vi "Gaussian surface with offset model.vi"(3 "output control":T1, 4 "data":variant, 5 "X":dbl[](array[numeric]), 6 "a":dbl[](array[numeric])) -> (0 "error out":errorcluster, 1 "f'(X,a)":dbl[][](array[numeric]), 2 "f(X,a)":dbl[](array[numeric]))   [LabVIEW 2023]
doc: "Gaussian surface with offset model"
uses:
  <vilib>/gmath/NumericalOptimization/LM_output select.ctl
  <vilib>/Utility/error.llb/Error Cluster From Error Code.vi
  <vilib>/Native 3D Graph/xcontrol/3DPC_SurfacePlot.xctl
  <vilib>/Native 3D Graph/classes/Base Datatype.lvclass
  <vilib>/ErrorRing/Error Ring.xnode
  <vilib>/gmath/NI_Gmath.lvlib
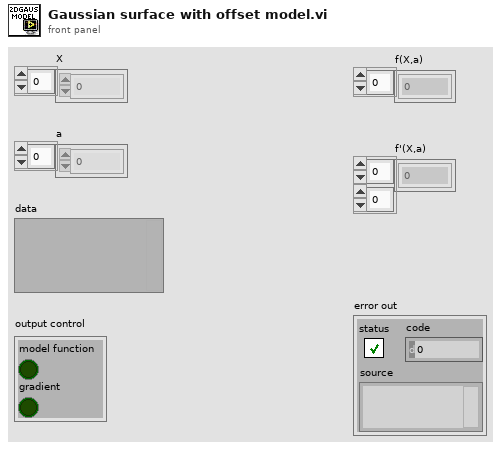
[diagram p1: front panel]
types:
  T1 = typedef "NI_Gmath.lvlib/LM_output select.ctl" = cluster{"model function":bool, "gradient":bool}
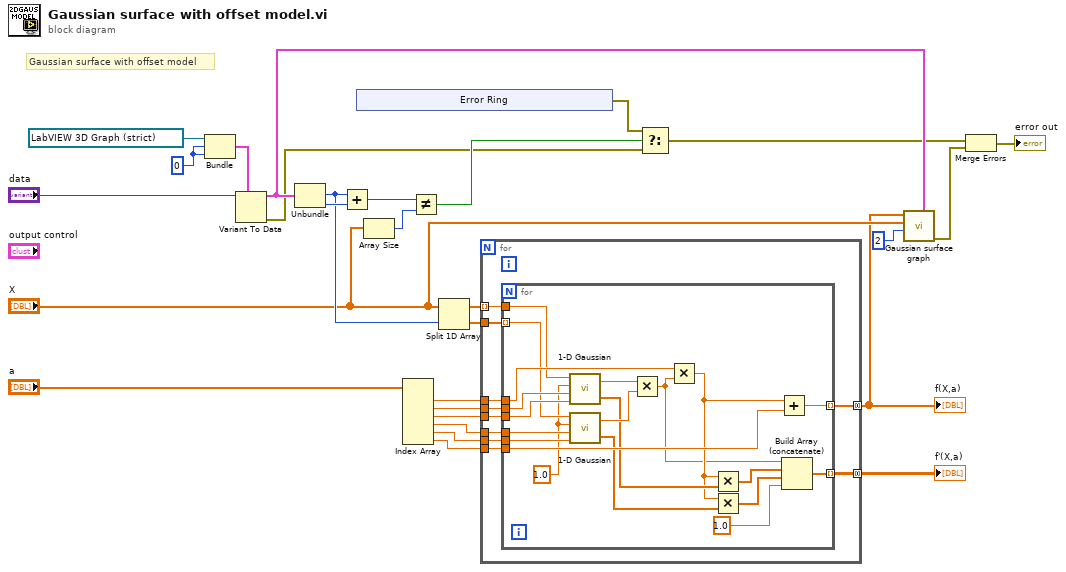
[diagram p0: block diagram]
diagram:
  w23 = 0
  # "Gaussian surface with offset model"
  n1 = Bundle("3D Surface Graph"=refnum<vi> refnum, w23, w23) -> (w15:cluster{"3D Surface Graph":refnum<vi>, i32, i32})  [unwired: 1 out]
  n2 = Variant To Data(type=w15, Variant="data") -> (data=w12:cluster{"3D Surface Graph":refnum<vi>, i32, i32}, error out=w5:errorcluster)  [unwired: 1 in]
  n3 = Unbundle(w12) -> (w13:i32, w14:i32)  [unwired: 1 out]
  n4 = Add(x=w13, y=w14) -> (x+y=w22:i32)
  n5 = xnode "Error Ring"() -> ("error out"=w8:errorcluster)
  n6 = Array Size(array="X") -> (size(s)=w21:i32)
  n7 = Index Array(array="a") -> (element #1=w28:dbl, element #2=w27:dbl, element #3=w26:dbl, element #4=w18:dbl, element #5=w17:dbl, element #6=w16:dbl)  [unwired: 6 in]
  n8 = Not Equal?(x=w22, y=w21) -> (x != y?=w9:bool)
  n9 = Split 1D Array(array="X", index=w13) -> (first subarray=w20:dbl[], second subarray=w19:dbl[])
  n10 = for {
    tunnel: w28 -> [w38]
    tunnel: w27 -> [w37]
    tunnel: w26 -> [w36]
    tunnel: w18 -> [w33]
    tunnel: w17 -> [w32]
    tunnel: w16 -> [w31]
    tunnel: w20 -> [w35] mode=indexing
    tunnel: w19 -> [w34]
    tunnel: [w30] -> w6 mode=concatenating
    tunnel: [w29] -> w3 mode=concatenating
    n11 = for {
      tunnel: [w57] -> w30 mode=indexing
      tunnel: w38 -> [w58]
      tunnel: w37 -> [w56]
      tunnel: w36 -> [w55]
      tunnel: w35 -> [w54]
      tunnel: w34 -> [w53] mode=indexing
      tunnel: w33 -> [w52]
      tunnel: w32 -> [w51]
      tunnel: w31 -> [w50]
      tunnel: [w46] -> w29 mode=indexing
      w49 = 1.0 ("a")
      n12 = call "1-D Gaussian.vi"("sigma"=w55, "m"=w56, "a"=w49, "x"=w54) -> ("y'"=w45:dbl[], "y"=w48:dbl)
      n13 = call "1-D Gaussian.vi"("sigma"=w51, "m"=w52, "a"=w49, "x"=w53) -> ("y'"=w43:dbl[], "y"=w47:dbl)
      n14 = Multiply(x=w48, y=w47) -> (x*y=w39:dbl)
      n15 = Multiply(x=w58, y=w39) -> (x*y=w40:dbl)
      n16 = Multiply(x=w40, y=w45) -> (x*y=w44:dbl[])
      n17 = Multiply(x=w40, y=w43) -> (x*y=w42:dbl[])
      n18 = Add(x=w40, y=w50) -> (x+y=w57:dbl)
      n19 = Build Array (concatenate)(w39, w44, w42, 1.0) -> (w46:dbl[])
    }
  }
  "f(X,a)" <- w6
  "f'(X,a)" <- w3
  n20 = Select(t=w8, s=w9, f=w5) -> (s? t:f=w7:errorcluster)
  n21 = call "Gaussian surface graph.vi"("output cluster"=w12, "plot number (1)"=2, "X"="X", "Y"=w6) -> ("error out"=w1:errorcluster)  [unwired: 7 out]
  n22 = Merge Errors(w7, w1) -> (→"error out":errorcluster)
